vi "Test_Rename_And_Set_Value.vi"   [LabVIEW 2025]
uses:
  8cebb4ce-4f0f-4319-9f7e-82e401bee674.vi
  0e244da9-745b-4f2d-a97c-0de3ccfbb071.vi
  57ba1f44-eecb-4af5-975d-0cda700306c1.vi
  Scripting Server.lvlib
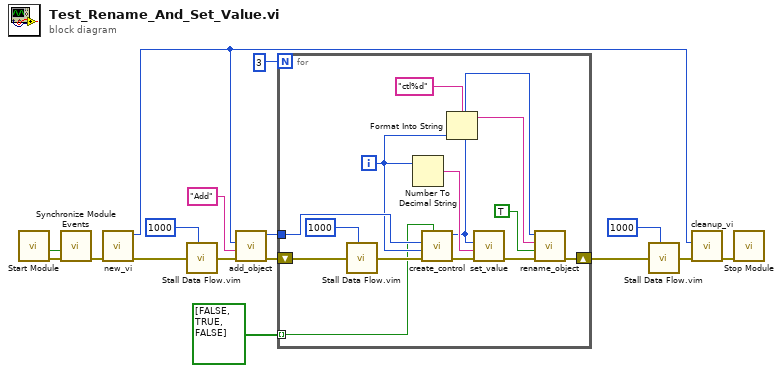
[diagram p0: block diagram]
diagram:
  n1 = call "Start Module.vi"() -> ("error out"=w15:errorcluster, "Wait for Event Sync?"=w16:bool)  [unwired: 7 in, 3 out]
  n2 = call "Synchronize Module Events.vi"("error in"=w15, "Wait for Event Sync?"=w16) -> ("error out"=w14:errorcluster)  [unwired: 9 in]
  n3 = call "new_vi.vi"("error in"=w14) -> ("error out"=w13:errorcluster, "vi_id"=w5:i32)  [unwired: 7 in, 2 out]
  n4 = call "Stall Data Flow.vim"("value in"=w13, "milliseconds to wait"=u32 1000) -> ("value out"=w12:errorcluster)  [unwired: 1 out]
  n5 = call "add_object.vi"("error in"=w12, "object_name"="Add", "vi_reference"=w5) -> ("error out"=w10:errorcluster, "object_id"=w9:i32)  [unwired: 5 in, 2 out]
  n6 = for {
    N: 3 -> [_]
    tunnel: w9 -> [w29]
    shift-right: [w23] -> w6
    shift-left: w10 -> [w30]
    tunnel: bool[] [FALSE, TRUE, FALSE] ("constant") -> [w17] mode=indexing
    i -> [w20]
    n7 = call "Stall Data Flow.vim"("value in"=w30, "milliseconds to wait"=u32 1000) -> ("value out"=w28:errorcluster)  [unwired: 1 out]
    n8 = Number To Decimal String(number=w20) -> (decimal integer string=w24:string)  [unwired: 1 in]
    n9 = call "create_control.vi"("constant"=w17, "error in"=w28, "terminal_index"=w20, "object_id"=w29) -> ("error out"=w26:errorcluster, "created_object_id"=w22:i32)  [unwired: 5 in, 1 out]
    n10 = Format Into String(format string="ctl%d", w20) -> (resulting string=w19:string)  [unwired: 2 in, 1 out]
    n11 = call "set_value.vi"("error in"=w26, "value"=w24, "object_id"=w22) -> ("error out"=w25:errorcluster)  [unwired: 7 in, 1 out]
    n12 = call "rename_object.vi"("error in"=w25, "label_visible"=TRUE, "new_label_name"=w19, "object_id"=w22) -> ("error out"=w23:errorcluster)  [unwired: 6 in, 1 out]
  }
  n13 = call "Stall Data Flow.vim"("value in"=w6, "milliseconds to wait"=u32 1000) -> ("value out"=w4:errorcluster)  [unwired: 1 out]
  n14 = call "cleanup_vi.vi"("error in"=w4, "vi_reference"=w5) -> ("error out"=w2:errorcluster)  [unwired: 7 in, 2 out]
  n15 = call "Stop Module.vi"("error in"=w2) -> ()  [unwired: 10 in, 1 out]
